vi "Read WS Message Broker Interface Ref.vi"(11 "Controller in":refnum<class "Controller.lvclass">) -> (2 "WS Message Broker Interface Ref.lvclass":refnum<class "WS Message Broker Interface Ref.lvclass">, 3 "Controller out":refnum<class "Controller.lvclass">)   [LabVIEW 2016, in "Controller Actor.lvlib" / "Controller.lvclass"]
uses:
  <userlib>/Common Components/Controller/Controller.lvclass
  <userlib>/Common Components/WebSocket Networking/WS Message Broker Interface Ref/WS Message Broker Interface Ref.lvclass
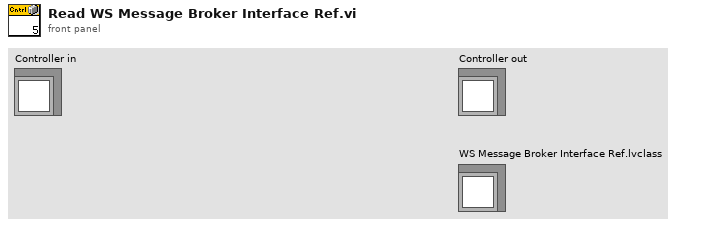
[diagram p1: front panel]
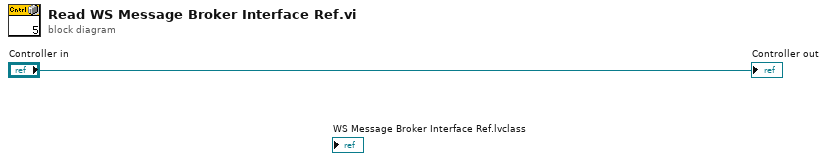
[diagram p0: block diagram]
diagram:
  "Controller out" <- "Controller in"
